vi "SubtractVI.vi"() -> ()   [LabVIEW 2019]
panel:
  out "Result":dbl
  in  "y":dbl
  in  "x":dbl
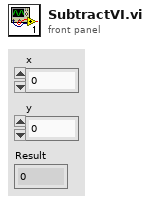
[diagram p1: front panel]
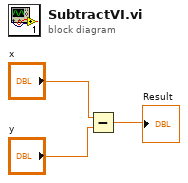
[diagram p0: block diagram]
diagram:
  n1 = Subtract(x="x", y="y") -> (x-y=→"Result":dbl)
